vi "Teleop.vi"(10 "Match Info":T1={"Autonomous Elapsed Seconds"=0.0, "TeleOp Elapsed Seconds"=0.0, "Disabled Elapsed Seconds"=0.0, "Visited Autonomous"=FALSE, "Visited TeleOp"=FALSE, "Visited Disabled"=FALSE, "Autonomous Settings"={"Autonomous Style"=enum."Independent", "VI Refnum"=refnum}}, 11 "Call Context":T2) -> ()   [LabVIEW 2012]
doc: "This VI is called for each TeleOp packet received from the DS where the robot is not disabled. It is often used to read from the joysticks and update I/O or to update setpoints for timed control loops. It should complete and return within 20 milliseconds or it may miss DS packets."
uses:
  <vilib>/Rock Robotics/WPI/DriverStation/WPI_DriverStationDerivedRobotMode.ctl
  <vilib>/Rock Robotics/WPI/DriverStation/WPI_DriverStationMatch Info.ctl
  <vilib>/Rock Robotics/WPI/Solenoid/WPI_SolenoidValue.ctl
  Robot Global Data.vi
  <vilib>/Rock Robotics/WPI/Joystick/WPI_JoystickGetSetRefNum.vi
  <vilib>/Rock Robotics/WPI/Solenoid/WPI_SolenoidSetEnum.vi
  <vilib>/Rock Robotics/WPI/RobotDrive/WPI_RobotDriveGetSetRefNum.vi
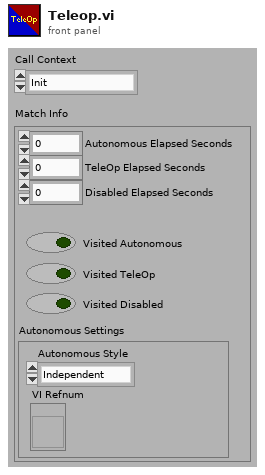
[diagram p1: front panel]
types:
  T1 = typedef "WPI_DriverStationMatch Info.ctl" = cluster{"Autonomous Elapsed Seconds":dbl, "TeleOp Elapsed Seconds":dbl, "Disabled Elapsed Seconds":dbl, "Visited Autonomous":bool, "Visited TeleOp":bool, "Visited Disabled":bool, "Autonomous Settings":cluster{"Autonomous Style":enum16{"Iterative", "Independent"}, "VI Refnum":refnum<vi>}}
  T2 = typedef "WPI_DriverStationDerivedRobotMode.ctl" = enum16{"Init", "Execute", "Stop"}
  T3 = typedef "WPI_JoystickDevRef.ctl" = cluster{"Device":T4}
  T4 = typedef "WPI_JoystickDeviceEnum.ctl" = enum16{"USB 1", "USB 2", "USB 3", "USB 4", "Kinect 1", "Kinect 2"}
  T5 = typedef "WPI_JoystickButtonState.ctl" = cluster{"Button 1":bool, "Button 2":bool, "Button 3":bool, "Button 4":bool, "Button 5":bool, "Button 6":bool, "Button 7":bool, "Button 8":bool, "Button 9":bool, "Button 10":bool, "Button 11":bool, "Button 12":bool}
  T6 = cluster{"axis 1 (x)":dbl, "axis 2 (y)":dbl, "axis 3 (throttle)":dbl, "axis 4":dbl, "axis 5":dbl, "axis 6":dbl}
  T7 = typedef "WPI_RobotDriveDevRef.ctl" = cluster{"DevStatus":errorcluster, "Motors[]":T8[], "Square Inputs":bool, "Max Output":dbl, "Isochronous":bool}
  T8 = typedef "WPI_MotorControlDeviceRef.ctl" = cluster{"DeviceStatus":errorcluster, "Type":enum16{"PWM", "CAN"}, "PWM":cluster{"Digital Module":T9, "PWM Channel":T10, "DeadBand":T11}, "CAN":cluster{"Device Number":u8, "Control Mode":T12, "Semaphore":T13, "Max Vout":dbl}, "Invert":bool, "TransformRef":T14, "InvTransformRef":T14}
  T9 = typedef "FPGA_TypedefDigitalModule.ctl" = enum16{"Digital Module 1", "Digital Module 2"}
  T10 = typedef "FPGA_DIOPWMChannel.ctl" = enum8{"PWM 1", "PWM 2", "PWM 3", "PWM 4", "PWM 5", "PWM 6", "PWM 7", "PWM 8", "PWM 9", "PWM 10", "Invalid"}
  T11 = typedef "WPI_PWMDeadband.ctl" = cluster{"Name":string, "maxPositivePwm":i32, "minPositivePwm":i32, "centerPwm":i32, "maxNegativePwm":i32, "minNegativePwm":i32, "angularRange":u16}
  T12 = typedef "WPI_CANJaguar_ControlMode.ctl" = enum8{"Percent VBus", "Current", "Speed", "Position", "Voltage"}
  T13 = typedef "Semaphore RefNum" = refnum<k1>
  T14 = typedef "WPI_PWMTransform_ConPane.ctl" = refnum<vi>
  T15 = typedef "WPI_ServoDeviceRef.ctl" = cluster{"DeviceStatus":errorcluster, "Digital Module":T9, "PWM Channel":T10, "DeadBand":T11}
  T16 = typedef "WPI_SolenoidValue.ctl" = enum16{"Off", "On", "Forward", "Reverse"}
  T17 = typedef "WPI_SolenoidDevRef.ctl" = cluster{"DevStatus":errorcluster, "Solenoid Module":T18, "Forward Solenoid Channel":T19, "Reverse Solenoid Channel":T19}
  T18 = typedef "FPGA_TypedefSolenoidModule.ctl" = enum16{"Solenoid Module 1", "Solenoid Module 2"}
  T19 = typedef "WPI_SolenoidChannel.ctl" = enum8{"Solenoid 1", "Solenoid 2", "Solenoid 3", "Solenoid 4", "Solenoid 5", "Solenoid 6", "Solenoid 7", "Solenoid 8", "Invalid"}
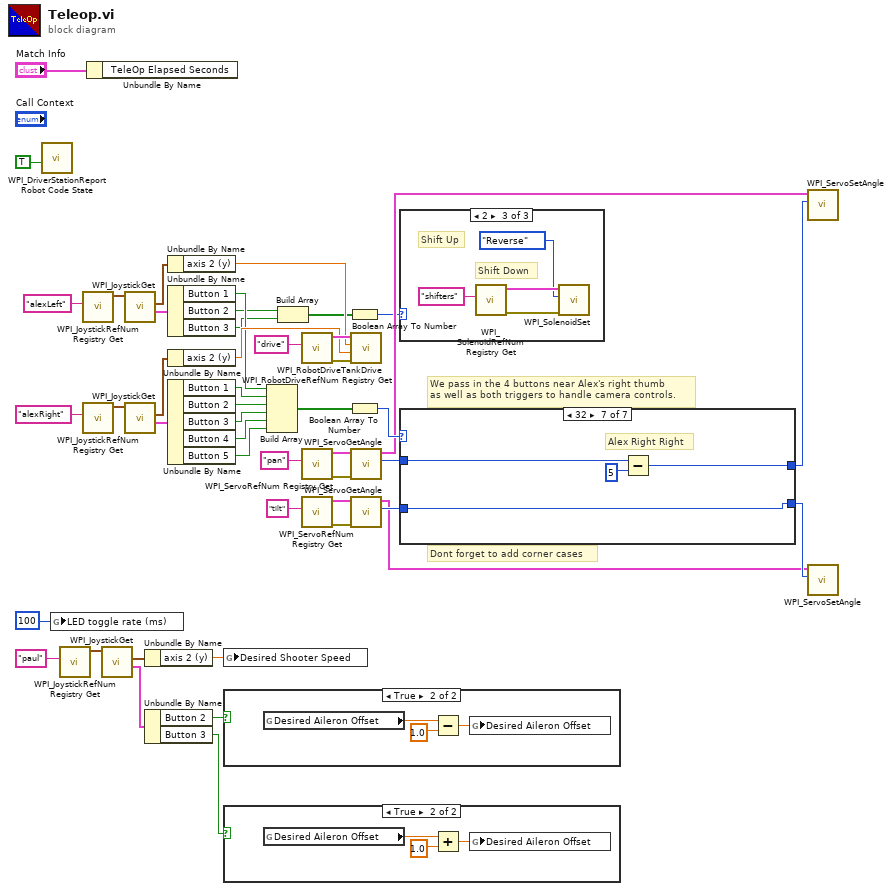
[diagram p0: block diagram]
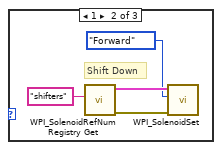
[diagram p3: hidden frame]
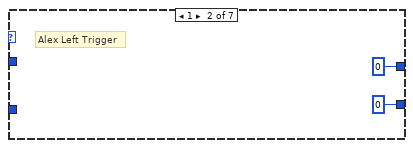
[diagram p5: hidden frame]
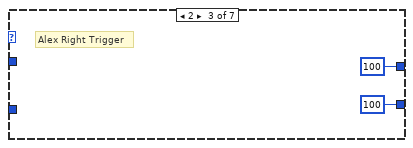
[diagram p6: hidden frame]
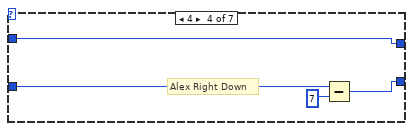
[diagram p7: hidden frame]
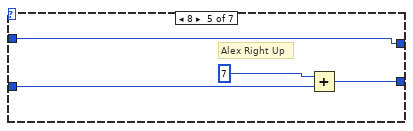
[diagram p8: hidden frame]
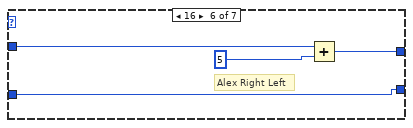
[diagram p9: hidden frame]
diagram:
  # "Dont forget to add corner cases"
  # "We pass in the 4 buttons near Alex's right thumb\nas well as both triggers to handle camera controls."
  n1 = call <vilib>:"WPI_DriverStationReport Robot Code State.vi"("TeleOp"=TRUE ("Autonomous")) -> ()  [unwired: 10 in, 1 out]
  n2 = global write "Robot Global Data.vi" "LED toggle rate (ms)"(u32 100 ("LED ms toggle rate")) -> ()
  n3 = call <vilib>:"WPI_JoystickRefNum Registry Get.vi"("refnum name"="paul") -> ("JoystickDevRef"=w31:T3)  [unwired: 9 in, 1 out]
  n4 = call <vilib>:"WPI_JoystickRefNum Registry Get.vi"("refnum name"="alexLeft") -> ("JoystickDevRef"=w41:T3)  [unwired: 9 in, 1 out]
  n5 = call <vilib>:"WPI_JoystickRefNum Registry Get.vi"("refnum name"="alexRight") -> ("JoystickDevRef"=w38:T3)  [unwired: 9 in, 1 out]
  n6 = Unbundle By Name("Match Info") -> ()  [unwired: 1 out]
  n7 = call <vilib>:"WPI_JoystickGet.vi"("JoystickDevRef"=w31) -> ("Buttons"=w29:T5, "Axes"=w33:T6)  [unwired: 4 in, 1 out]
  n8 = call <vilib>:"WPI_JoystickGet.vi"("JoystickDevRef"=w41) -> ("Buttons"=w19:T5, "Axes"=w36:T6)  [unwired: 4 in, 1 out]
  n9 = call <vilib>:"WPI_JoystickGet.vi"("JoystickDevRef"=w38) -> ("Buttons"=w26:T5, "Axes"=w37:T6)  [unwired: 4 in, 1 out]
  n10 = Unbundle By Name(w33) -> ("axis 2 (y)"=w30:dbl)
  n11 = Unbundle By Name(w29) -> ("Button 2"=w28:bool, "Button 3"=w27:bool)
  n12 = Unbundle By Name(w36) -> ("axis 2 (y)"=w35:dbl)
  n13 = Unbundle By Name(w19) -> ("Button 1"=w18:bool, "Button 2"=w3:bool, "Button 3"=w2:bool)
  n14 = Unbundle By Name(w37) -> ("axis 2 (y)"=w34:dbl)
  n15 = Unbundle By Name(w26) -> ("Button 1"=w17:bool, "Button 2"=w25:bool, "Button 3"=w24:bool, "Button 4"=w23:bool, "Button 5"=w22:bool)
  n16 = global write "Robot Global Data.vi" "Desired Shooter Speed"(w30) -> ()
  n17 = case shown="True" w28 {
    frame False {
    }
    frame True {
      n18 = global read "Robot Global Data.vi" "Desired Aileron Offset"() -> (w50:dbl)
      n19 = Subtract(x=w50, y=1.0) -> (x-y=w48:dbl)
      n20 = global write "Robot Global Data.vi" "Desired Aileron Offset"(w48) -> ()
    }
  }
  n21 = case shown="True" w27 {
    frame False {
    }
    frame True {
      n22 = global read "Robot Global Data.vi" "Desired Aileron Offset"() -> (w53:dbl)
      n23 = Add(x=w53, y=1.0) -> (x+y=w51:dbl)
      n24 = global write "Robot Global Data.vi" "Desired Aileron Offset"(w51) -> ()
    }
  }
  n25 = Build Array(w18, w17, w25, w24, w23, w22) -> (w21:bool[])
  n26 = Build Array(w3, w2) -> (w4:bool[])
  n27 = call <vilib>:"WPI_RobotDriveRefNum Registry Get.vi"("refnum name"="drive") -> ("error out"=w42:errorcluster, "RobotDriveDevRef"=w44:T7)  [unwired: 9 in]
  n28 = call <vilib>:"WPI_ServoRefNum Registry Get.vi"("refnum name"="pan") -> ("error out"=w16:errorcluster, "ServoDeviceRef"=w15:T15)  [unwired: 9 in]
  n29 = call <vilib>:"WPI_ServoRefNum Registry Get.vi"("refnum name"="tilt") -> ("error out"=w11:errorcluster, "ServoDeviceRef"=w12:T15)  [unwired: 9 in]
  n30 = Boolean Array To Number(Boolean array=w4) -> (number=w1:u32)
  n31 = Boolean Array To Number(Boolean array=w21) -> (number=w20:u32)
  n32 = call <vilib>:"WPI_RobotDriveTankDrive.vi"("error in (no error)"=w42, "Right axis value"=w34, "Left axis value"=w35, "RobotDriveDevRef"=w44) -> ()  [unwired: 5 in, 3 out]
  n33 = call <vilib>:"WPI_ServoGetAngle.vi"("ServoDeviceRef"=w15, "error in (no error)"=w16) -> ("ServoDeviceRef"=w8:T15, "Angle"=w10:u16)  [unwired: 6 in, 1 out]
  n34 = call <vilib>:"WPI_ServoGetAngle.vi"("ServoDeviceRef"=w12, "error in (no error)"=w11) -> ("ServoDeviceRef"=w5:T15, "Angle"=w9:u16)  [unwired: 6 in, 1 out]
  n35 = case shown="2" w1 {
    frame 0, Default {
    }
    frame 1 {
      # "Shift Down"
      n36 = call <vilib>:"WPI_SolenoidRefNum Registry Get.vi"("refnum name"="shifters") -> ("error out"=w56:errorcluster, "SolenoidDevRef"=w55:T17)  [unwired: 9 in]
      n37 = call-poly <vilib>:"WPI_SolenoidSet.vi"("error in (no error)"=w56, "Value"=WPI_SolenoidValue."Forward", "SolenoidDevRef"=w55) -> ()  [unwired: 7 in, 2 out]
    }
    frame 2 {
      # "Shift Down"
      # "Shift Up"
      n38 = call <vilib>:"WPI_SolenoidRefNum Registry Get.vi"("refnum name"="shifters") -> ("error out"=w60:errorcluster, "SolenoidDevRef"=w59:T17)  [unwired: 9 in]
      n39 = call-poly <vilib>:"WPI_SolenoidSet.vi"("error in (no error)"=w60, "Value"=WPI_SolenoidValue."Reverse", "SolenoidDevRef"=w59) -> ()  [unwired: 7 in, 2 out]
    }
  }
  n40 = case shown="32" w20 {
    tunnel: w10 -> [w63 _ _ w71 w75 w79 w80]
    tunnel: w9 -> [w62 _ _ w70 w74 w78 w83]
    tunnel: [w63 u16 0 ("Angle") u16 100 ("Angle") w71 w75 w77 w82] -> w7
    tunnel: [w62 u16 0 ("Angle") u16 100 ("Angle") w69 w73 w78 w83] -> w6
    frame 0, Default {
      # "No Camera Control Changes"
    }
    frame 1 {
      # "Alex Left Trigger"
    }
    frame 2 {
      # "Alex Right Trigger"
    }
    frame 4 {
      # "Alex Right Down"
      n41 = Subtract(x=w70, y=u16 7) -> (x-y=w69:u16)
    }
    frame 8 {
      # "Alex Right Up"
      n42 = Add(x=u16 7, y=w74) -> (x+y=w73:u16)
    }
    frame 16 {
      # "Alex Right Left"
      n43 = Add(x=w79, y=u16 5) -> (x+y=w77:u16)
    }
    frame 32 {
      # "Alex Right Right"
      n44 = Subtract(x=w80, y=u16 5 ("x")) -> (x-y=w82:u16)
    }
  }
  n45 = call <vilib>:"WPI_ServoSetAngle.vi"("Angle"=w7, "ServoDeviceRef"=w8) -> ()  [unwired: 8 in, 2 out]
  n46 = call <vilib>:"WPI_ServoSetAngle.vi"("Angle"=w6, "ServoDeviceRef"=w5) -> ()  [unwired: 8 in, 2 out]
